vi "NodosDePropiedad.vi"() -> ()   [LabVIEW 2020]
panel:
  in  "stop":bool
  in  "Limite muestreo":i32
  in  "Limite superior":dbl
  in  "Numeric":dbl
  out "No. Muestreo":i32
  out "String":string
  out "Fuera de rango":bool
  out "Temperatura":cluster{dbl, "Limite superior":dbl}(graph)
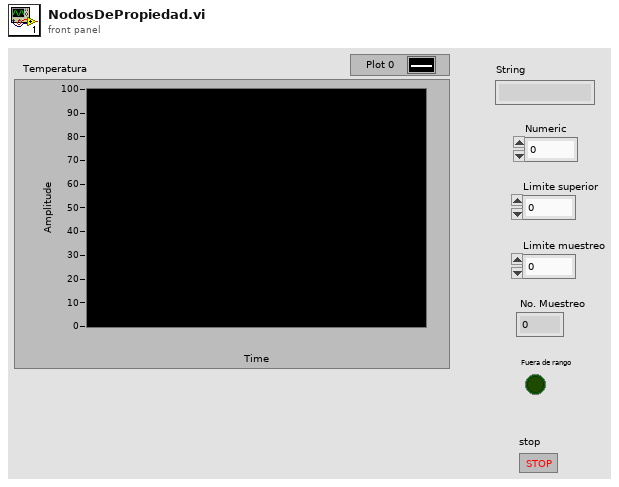
[diagram p1: front panel]
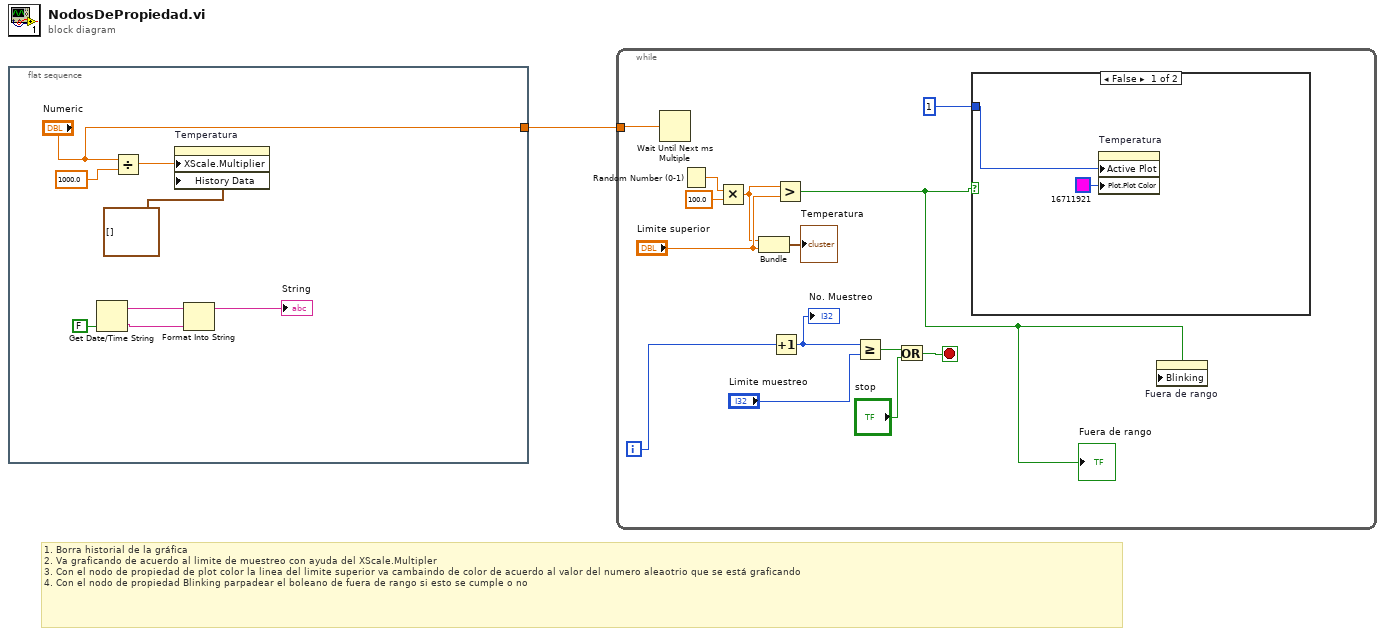
[diagram p0: block diagram]
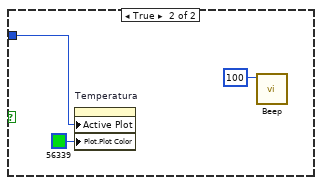
[diagram p2: hidden frame]
diagram:
  # "1. Borra historial de la gráfica\n2. Va graficando de acuerdo al limite de muestreo con ayuda del XScale.Multipler\n3. Con el nodo de propiedad de plot color la linea del limite superior va cambaindo de color de acuerdo al valor del numero aleaotrio que se está graficando\n4. Con el nodo de propiedad Blinking parpadear el boleano de fuera de rango si esto se cumple o no"
  n1 = flat-sequence {
    tunnel: ["Numeric"] -> w1
    frame #0 {
      n2 = Get Date/Time String(want seconds? (F)=FALSE) -> (date string=w8:string, time string=w7:string)  [unwired: 2 in]
      n3 = Divide(x="Numeric", y=1000.0) -> (x/y=w5:dbl)
      n4 = property on="Temperatura" class="WFChart (strict)"("XScale.Multiplier"=w5, "History Data"=cluster{dbl, "Limite superior":dbl}[] []) -> ()  [unwired: 2 in, 2 out]
      n5 = Format Into String(initial string=w8, w7) -> (resulting string=→"String":string)  [unwired: 2 in, 1 out]
    }
  }
  n6 = while {
    tunnel: w1 -> [w23]
    i -> [w17]
    stop <- w13 stop-if-true
    n7 = Wait Until Next ms Multiple(millisecond multiple=w23) -> ()  [unwired: 1 out]
    n8 = Random Number (0-1)() -> (number: 0 to 1=w22:dbl)
    n9 = Multiply(x=w22, y=100.0) -> (x*y=w19:dbl)
    n10 = Bundle(w19, "Limite superior"="Limite superior") -> (→"Temperatura":cluster{dbl, "Limite superior":dbl})  [unwired: 1 in]
    n11 = Increment(x=w17) -> (x+1=w15:i32)
    "No. Muestreo" <- w15
    n12 = Greater?(x=w19, y="Limite superior") -> (0:w11:bool)
    "Fuera de rango" <- w11
    n13 = Greater Or Equal?(x=w15, y="Limite muestreo") -> (x >= y?=w16:bool)
    n14 = Or(x=w16, y="stop") -> (x .or. y?=w13:bool)
    n15 = case shown="False" w11 {
      tunnel: u32 1 ("Active Plot") -> [w24 w27]
      frame False {
        n16 = property on="Temperatura" class="WFChart (strict)"("Active Plot"=w24, "Plot.Plot Color"=u32 16711921) -> ()  [unwired: 2 in, 2 out]
      }
      frame True {
        n17 = property on="Temperatura" class="WFChart (strict)"("Active Plot"=w27, "Plot.Plot Color"=u32 56339) -> ()  [unwired: 2 in, 2 out]
        n18 = call <vilib>:"Beep.vi"("frequency (Hz)"=u32 100) -> ()  [unwired: 11 in]
      }
    }
    n19 = property on="Fuera de rango" class="Bool (strict)"("Blinking"=w11) -> ()  [unwired: 2 in, 2 out]
  }
